vi "Parse ERD Read Results.vi"(0 "Verify ERD Response?":bool=TRUE, 2 "Read ERD List":T2[](array[typedef]) {"ERD Number" format="%.0x"}, 5 "Raw Message":string, 7 "Converted Data":T4 {"CRC" format="%04x"; "Length" format="%02x"; "Command" format="%02x"; "Destination" format="%02x"; "Source" format="%02x"}, 11 "Error In":errorcluster) -> (4 "Pass/Fail?":bool, 8 "ERD Data Out":T1[](array[typedef]) {"ERD Number" format="%.0x"}, 15 "Error Out":errorcluster)   [LabVIEW 2020, in "GEA2_Toolkit.lvlib"]
doc: "This VI takes the converted return data from the GEA2 Send and Receive and formats the Data based on the selections made in the Read ERD list. In addition, it also verifies the ERDs requested were returned."
uses:
  library/GEA2_Toolkit.lvlib
  type defs/Data Out.ctl
  type defs/ERD Read Data In.ctl
  type defs/Data Type.ctl
  type defs/ERD Read Data Out.ctl
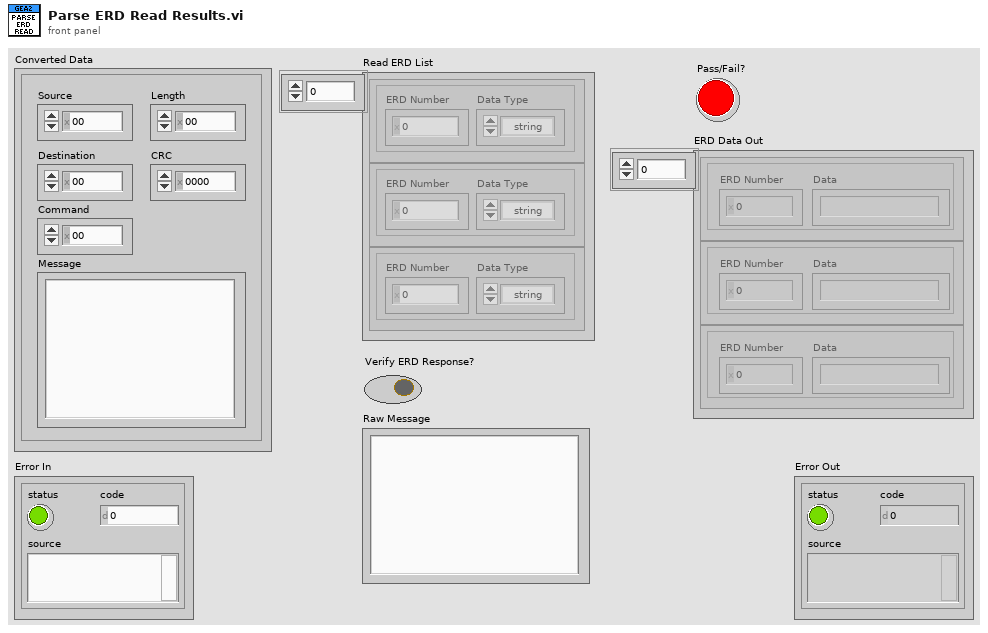
[diagram p1: front panel]
types:
  T1 = typedef "GEA2_Toolkit.lvlib/ERD Read Data Out.ctl" = cluster{"ERD Number":u16, "Data":string}
  T2 = typedef "GEA2_Toolkit.lvlib/ERD Read Data In.ctl" = cluster{"ERD Number":u16, "Data Type":T3}
  T3 = typedef "GEA2_Toolkit.lvlib/Data Type.ctl" = enum16{"string", "boolean", "uint8_t", "uint16_t", "uint32_t", "uint64_t", "int8_t", "int16_t", "int32_t", "int64_t"}
  T4 = typedef "GEA2_Toolkit.lvlib/Data Out.ctl" = cluster{"Source":u8, "Destination":u8, "Command":u8, "Length":u8, "CRC":u16, "Message":string}
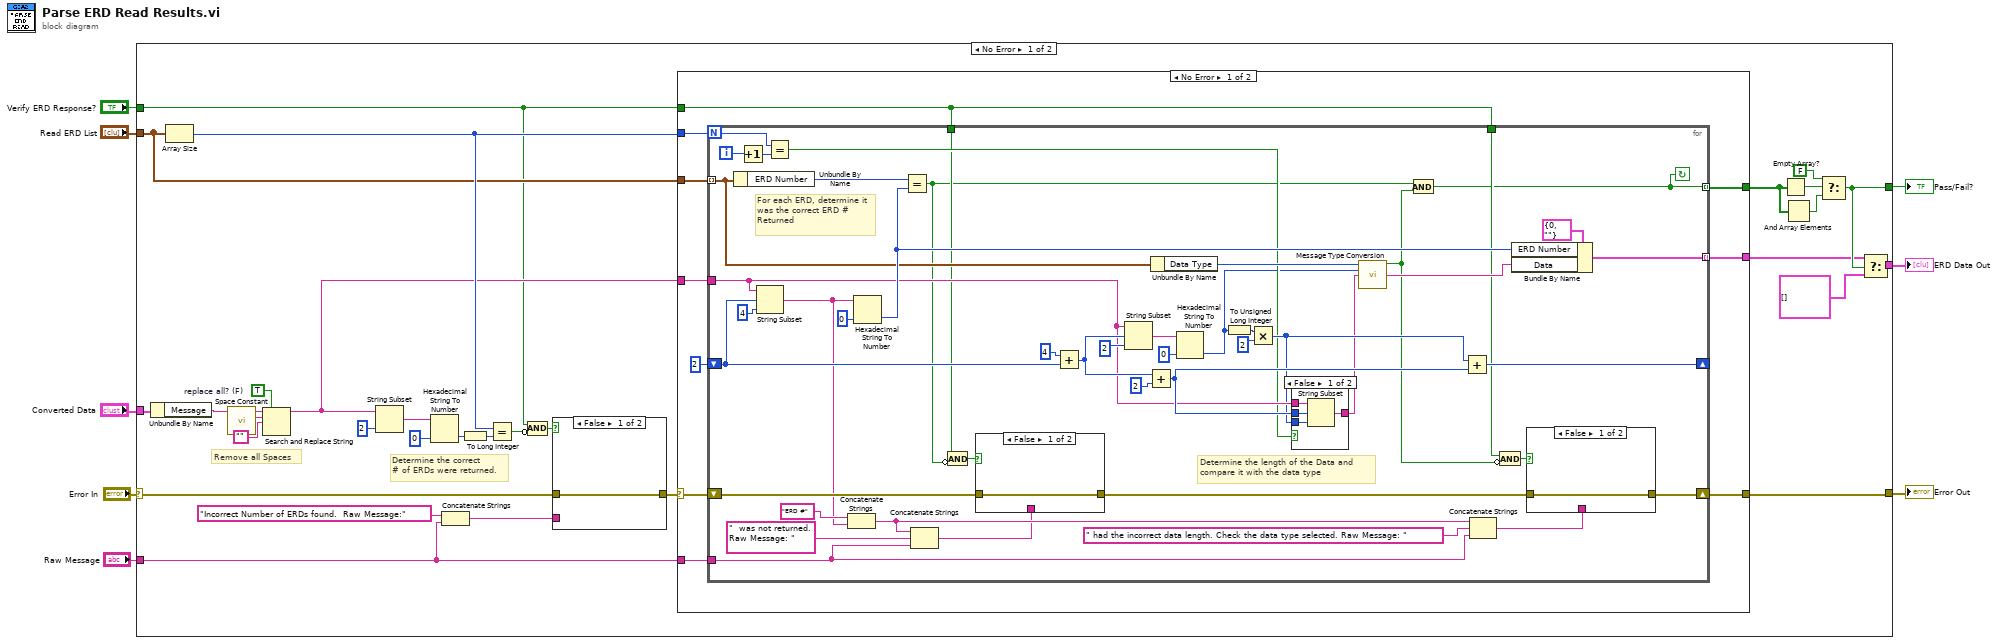
[diagram p0: block diagram]
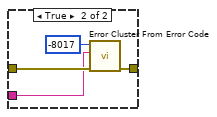
[diagram p2: hidden frame]
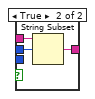
[diagram p3: hidden frame]
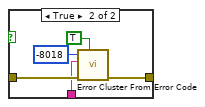
[diagram p4: hidden frame]
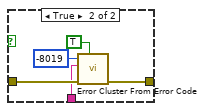
[diagram p5: hidden frame]
diagram:
  n1 = case shown="No Error" "Error In" {
    selector: "Error In" -> [w16 w120]
    tunnel: "Converted Data" -> [w38 _]
    tunnel: "Read ERD List" -> [w31 _]
    tunnel: [w26 _] -> w6
    tunnel: [w23 _] -> w5
    tunnel: [w17 w120] -> w3
    tunnel: "Raw Message" -> [w12 _]
    tunnel: "Verify ERD Response?" -> [w11 _]
    frame No Error {
      w18 = TRUE  # replace all? (F)
      # "Remove all Spaces"
      # "Determine the correct \n# of ERDs were returned."
      n2 = Unbundle By Name(w38) -> ("Message"=w20:string)
      n3 = Array Size(array=w31) -> (size(s)=w34:i32)
      n4 = call <vilib>:"Space Constant.vi"() -> ("String"=w22:string)
      n5 = Search and Replace String(replace all?=w18, input string=w20, search string=w22, replace string="") -> (result string=w19:string)  [unwired: 4 in, 3 out]
      n6 = String Subset(string=w19, length (rest)=2 ("length (rest)")) -> (substring=w36:string)  [unwired: 1 in]
      n7 = Hexadecimal String To Number(string=w36, default (0uL)=u8 0) -> (number=w32:u8)  [unwired: 1 in, 1 out]
      n8 = Concatenate Strings("Incorrect Number of ERDs found.  Raw Message:" ("string"), w12) -> (w14:string)
      n9 = To Long Integer(number=w32) -> (32bit integer=w33:i32)
      n10 = Equal?(x=w34, y=w33) -> (x = y?=w10:bool)
      n11 = Compound Arithmetic op=AND(w11, invert w10) -> (w9:bool)
      n12 = case shown="False" w9 {
        tunnel: [w39 w43] -> w13
        tunnel: w16 -> [w39 w41]
        tunnel: w14 -> [_ w40]
        frame False {
        }
        frame True {
          n13 = call <vilib>:"Error Cluster From Error Code.vi"("error in (no error)"=w41, "error message (\"\")"=w40, "error code (0)"=-8017) -> ("error out"=w43:errorcluster)  [unwired: 6 in]
        }
      }
      n14 = case shown="No Error" w13 {
        selector: w13 -> [w47 w119]
        tunnel: w34 -> [w53 _]
        tunnel: [w49 _] -> w30
        tunnel: w19 -> [w52 _]
        tunnel: w31 -> [w51 _]
        tunnel: [w50 _] -> w25
        tunnel: [w48 w119] -> w17
        tunnel: w12 -> [w46 _]
        tunnel: w11 -> [w44 _]
        frame No Error {
          n15 = for {
            N: w53 -> [w65]
            tunnel: w52 -> [w67]
            shift-right: [w83] -> _
            shift-left: u32 2 -> [w84]
            tunnel: w51 -> [w87] mode=indexing
            tunnel: [w96] -> w50 mode=indexing
            tunnel: [w54] -> w49 mode=indexing
            shift-right: [w92] -> w48
            shift-left: w47 -> [w89]
            tunnel: w46 -> [w76]
            tunnel: w44 -> [w61]
            tunnel: w44 -> [w57]
            i -> [w91]
            stop <- w54 continue-if-true
            # "For each ERD, determine it was the correct ERD # Returned"
            # "Determine the length of the Data and\ncompare it with the data type"
            n16 = Unbundle By Name(w87) -> ("ERD Number"=w95:u16)
            n17 = Increment(x=w91) -> (x+1=w90:i32)
            n18 = String Subset(string=w67, offset (0)=w84, length (rest)=4 ("length (rest)")) -> (substring=w81:string)
            n19 = Equal?(x=w65, y=w90) -> (x = y?=w64:bool)
            n20 = Concatenate Strings("ERD #" ("string"), w81) -> (w79:string)
            n21 = Hexadecimal String To Number(string=w81, default (0uL)=u16 0) -> (number=w94:u16)  [unwired: 1 in, 1 out]
            n22 = Equal?(x=w95, y=w94) -> (x = y?=w60:bool)
            n23 = Concatenate Strings(w79, "  was not returned. Raw Message: " ("string"), w76) -> (w77:string)
            n24 = Compound Arithmetic op=AND(w61, invert w60) -> (w62:bool)
            n25 = case shown="False" w62 {
              tunnel: [w107 w112] -> w88
              tunnel: w89 -> [w107 w111]
              tunnel: w77 -> [_ w108]
              frame False {
              }
              frame True {
                n26 = call <vilib>:"Error Cluster From Error Code.vi"("show call chain? (False)"=TRUE, "error in (no error)"=w111, "error message (\"\")"=w108, "error code (0)"=-8018) -> ("error out"=w112:errorcluster)  [unwired: 5 in]
              }
            }
            n27 = Add(x=u32 4, y=w84) -> (x+y=w69:u32)
            n28 = String Subset(string=w67, offset (0)=w69, length (rest)=2 ("length (rest)")) -> (substring=w73:string)
            n29 = Add(x=w69, y=u32 2) -> (x+y=w68:u32)
            n30 = Unbundle By Name(w87) -> ("Data Type"=w86:T3)
            n31 = Hexadecimal String To Number(string=w73, default (0uL)=u8 0 ("default (0 U32)")) -> (number=w55:u8)  [unwired: 1 in, 1 out]
            n32 = To Unsigned Long Integer(number=w55) -> (unsigned 32bit integer=w56:u32)
            n33 = Multiply(x=w56, y=u32 2) -> (x*y=w66:u32)
            n34 = case shown="False" w64 {
              tunnel: w67 -> [w103 w106]
              tunnel: w68 -> [w101 w105]
              tunnel: [w102 w104] -> w63
              tunnel: w66 -> [w100 _]
              frame False {
                n35 = String Subset(string=w103, offset (0)=w101, length (rest)=w100) -> (substring=w102:string)
              }
              frame True {
                n36 = String Subset(string=w106, offset (0)=w105) -> (substring=w104:string)  [unwired: 1 in]
              }
            }
            n37 = call "Message Type Conversion.vi"("Data Type"=w86, "Data Length"=w55, "Message In"=w63) -> ("Pass/Fail?"=w59:bool, "Message Out"=w93:string)  [unwired: 11 in]
            n38 = And(x=w60, y=w59) -> (x .and. y?=w54:bool)
            n39 = Add(x=w66, y=w68) -> (x+y=w83:u32)
            n40 = Concatenate Strings(w79, " had the incorrect data length. Check the data type selected. Raw Message: " ("string"), w76) -> (w75:string)
            n41 = Compound Arithmetic op=AND(w57, invert w59) -> (w58:bool)
            n42 = Bundle By Name(cluster=T1 {"ERD Number"=0, "Data"=""} ("ERD Output"), "ERD Number"=w94, "Data"=w93) -> (w96:T1)
            n43 = case shown="False" w58 {
              tunnel: [w113 w118] -> w92
              tunnel: w88 -> [w113 w117]
              tunnel: w75 -> [_ w114]
              frame False {
              }
              frame True {
                n44 = call <vilib>:"Error Cluster From Error Code.vi"("show call chain? (False)"=TRUE, "error in (no error)"=w117, "error message (\"\")"=w114, "error code (0)"=-8019) -> ("error out"=w118:errorcluster)  [unwired: 5 in]
              }
            }
          }
        }
        frame Error {
        }
      }
      n45 = Empty Array?(array=w30) -> (empty?=w29:bool)
      n46 = And Array Elements(Boolean array=w30) -> (logical AND=w28:bool)
      n47 = Select(t=FALSE, s=w29, f=w28) -> (s? t:f=w26:bool)
      n48 = Select(t=w25, s=w26, f=T1[] []) -> (s? t:f=w23:T1[])
    }
    frame Error {
    }
  }
  "Pass/Fail?" <- w6
  "ERD Data Out" <- w5
  "Error Out" <- w3
